vi "Proposed_Interface.vi"() -> ()   [LabVIEW 2020]
panel:
  out "?":T1
  out "?":T2
  out "?":T3
  out "?":T4
  out "?":T5
  out "?":T5
  out "?":T6
  out "?":T6
  out "?":T7
  out "?":T8
  out "?":T9
  out "?":T10
  out "Led":T11
  in  "Traffic info":T12
  # "Vehicel count will be incresed manually right now, \nbut for RFID it should detect on its own."
  # "If same RFID is detected twice, the RFID detection error \nwill increase and count of vehicles will decrease."
  # "Speeding vehicle,."
  # "Concentrate more on emergency vehicle detection."
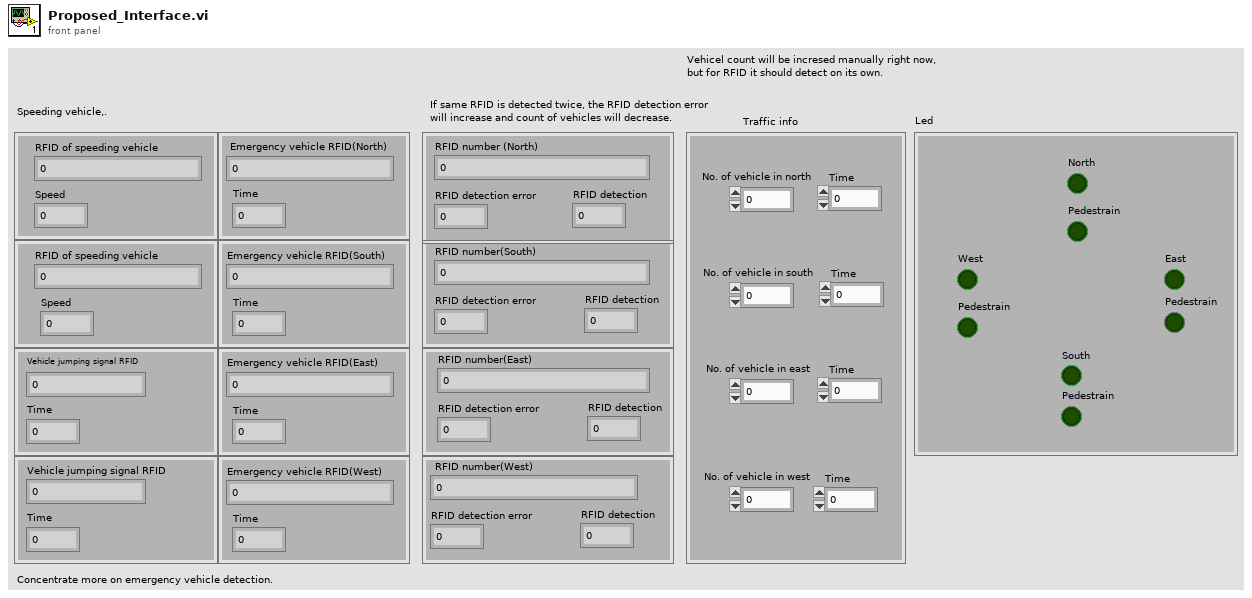
[diagram p1: front panel]
types:
  T1 = cluster{"Emergency vehicle RFID(West)":dbl, "Time":dbl}
  T2 = cluster{"Emergency vehicle RFID(East)":dbl, "Time":dbl}
  T3 = cluster{"Emergency vehicle RFID(South)":dbl, "Time":dbl}
  T4 = cluster{" Emergency vehicle RFID(North)":dbl, "Time":dbl}
  T5 = cluster{"RFID of speeding vehicle":dbl, "Speed":dbl}
  T6 = cluster{"Vehicle jumping signal RFID":dbl, "Time":dbl}
  T7 = cluster{"RFID number(West)":dbl, "RFID detection error":dbl, "RFID detection":dbl}
  T8 = cluster{"RFID number(South)":dbl, "RFID detection error":dbl, "RFID detection":dbl}
  T9 = cluster{"RFID number(East)":dbl, "RFID detection error":dbl, "RFID detection":dbl}
  T10 = cluster{"RFID number (North)":dbl, "RFID detection error":dbl, "RFID detection":dbl}
  T11 = cluster{"North":bool, "East":bool, "South":bool, "West":bool, "Pedestrain":bool, "Pedestrain":bool, "Pedestrain":bool, "Pedestrain":bool}
  T12 = cluster{"No. of vehicle in north":dbl, "No. of vehicle in east":dbl, "Time ":dbl, "No. of vehicle in south":dbl, "Time":dbl, "No. of vehicle in west":dbl, "Time":dbl, "Time":dbl}
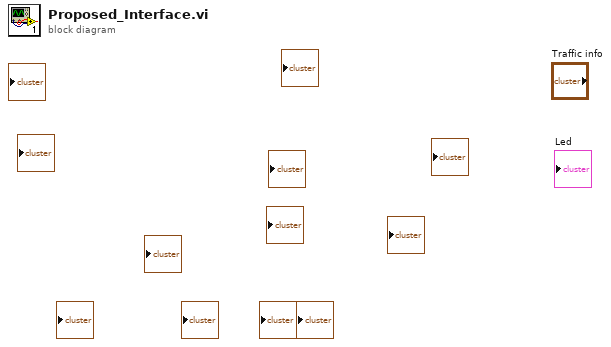
[diagram p0: block diagram]
diagram:
